vi "BuildG#ReleaseZip.vi"() -> ()   [LabVIEW 2012]
panel:
  out "error out":errorcluster
  in  "G# Package":string="G# Framework 1.7.0"
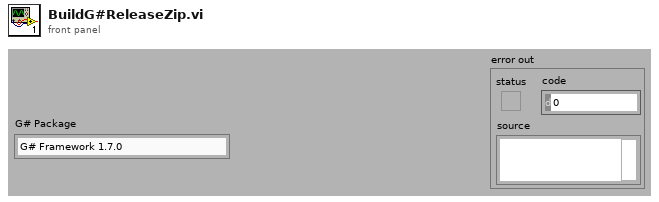
[diagram p1: front panel]
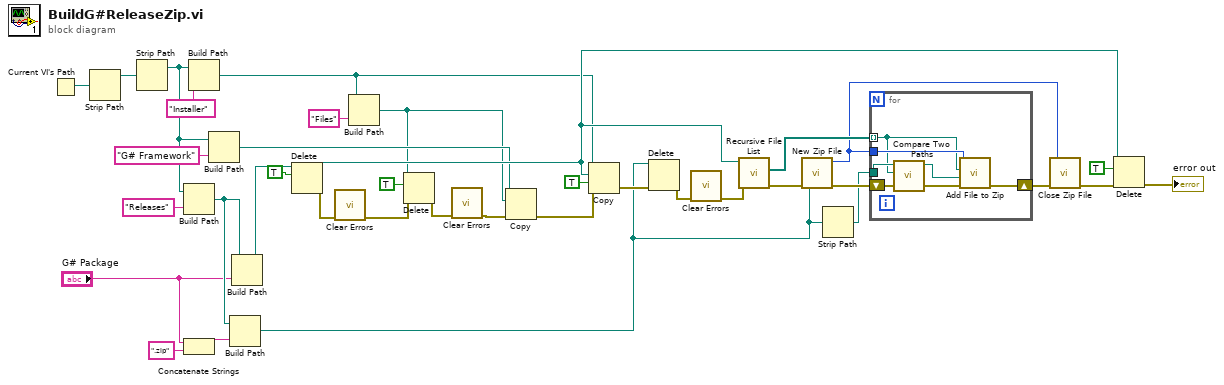
[diagram p0: block diagram]
diagram:
  n1 = Current VI's Path() -> (path=w37:path)
  n2 = Strip Path(path=w37) -> (stripped path=w36:path)  [unwired: 1 out]
  n3 = Strip Path(path=w36) -> (stripped path=w11:path)  [unwired: 1 out]
  n4 = Build Path(base path=w11, name or relative path="Releases") -> (appended path=w30:path)
  n5 = Concatenate Strings("G# Package", ".zip" ("string")) -> (w29:string)
  n6 = Build Path(base path=w11, name or relative path="Installer") -> (appended path=w8:path)
  n7 = Build Path(base path=w11, name or relative path="G# Framework") -> (appended path=w3:path)
  n8 = Build Path(base path=w30, name or relative path=w29) -> (appended path=w19:path)
  n9 = Build Path(base path=w30, name or relative path="G# Package") -> (appended path=w31:path)
  n10 = Delete(path (use dialog)=w31, entire hierarchy (F)=TRUE) -> (deleted path=w13:path, error out=w18:errorcluster)  [unwired: 3 in, 1 out]
  n11 = call <vilib>:"Clear Errors.vi"("error in (no error)"=w18) -> ("error out"=w9:errorcluster)  [unwired: 6 in]
  n12 = Build Path(base path=w8, name or relative path="Files") -> (appended path=w2:path)
  n13 = Delete(path (use dialog)=w2, entire hierarchy (F)=TRUE, error in=w9) -> (error out=w5:errorcluster)  [unwired: 2 in, 2 out]
  n14 = call <vilib>:"Clear Errors.vi"("error in (no error)"=w5) -> ("error out"=w4:errorcluster)  [unwired: 6 in]
  n15 = Copy(8:w4, 10:w2, 11:w3) -> (0:w1:errorcluster)  [unwired: 2 in, 2 out]
  n16 = Copy(8:w1, 9:TRUE ("overwrite (F)"), 10:w13, 11:w8) -> (0:w26:errorcluster)  [unwired: 1 in, 2 out]
  n17 = Delete(path (use dialog)=w19, error in=w26) -> (error out=w17:errorcluster)  [unwired: 3 in, 2 out]
  n18 = call <vilib>:"Clear Errors.vi"("error in (no error)"=w17) -> ("error out"=w16:errorcluster)  [unwired: 6 in]
  n19 = call <vilib>:"Recursive File List.vi"("error in (no error)"=w16, "Folder Path"=w13) -> ("error out"=w24:errorcluster, "All Files in Dir"=w23:path[])  [unwired: 5 in, 3 out]
  n20 = call <vilib>:"New Zip File.vi"("error in (no error)"=w24, "target"=w19) -> ("error out"=w25:errorcluster, "zip file out"=w20:i64)  [unwired: 3 in, 1 out]
  n21 = Strip Path(path=w19) -> (stripped path=w22:path)  [unwired: 1 out]
  n22 = for {
    tunnel: w20 -> [w43]
    shift-right: [w44] -> w21
    shift-left: w25 -> [w42]
    tunnel: w23 -> [w39] mode=indexing
    tunnel: w22 -> [w40]
    n23 = call <vilib>:"Compare Two Paths.vi"("error in (no error)"=w42, "Path 2"=w39, "Path 1"=w40) -> ("error out"=w41:errorcluster, "Relative Path from 1 to 2"=w38:path)  [unwired: 5 in, 2 out]
    n24 = call <vilib>:"Add File to Zip.vi"("error in (no error)"=w41, "destination path in zip"=w38, "source file path"=w39, "zip file in"=w43) -> ("error out"=w44:errorcluster)  [unwired: 6 in, 1 out]
  }
  n25 = call <vilib>:"Close Zip File.vi"("error in (no error)"=w21, "zip file in"=w20) -> ("error out"=w15:errorcluster)  [unwired: 5 in]
  n26 = Delete(path (use dialog)=w13, entire hierarchy (F)=TRUE, error in=w15) -> (error out=→"error out":errorcluster)  [unwired: 2 in, 2 out]
